vi "Construct.vi"(8 "error in (no error)":errorcluster, 9 "Ordered deps":refnum<class "ProjectItem.lvclass">[](array[class]), 10 "Application in":refnum<vi>, 11 "BuildManager in":refnum<class "BuildManager.lvclass">) -> (0 "error out":errorcluster, 3 "BuildManager out":refnum<class "BuildManager.lvclass">)   [LabVIEW 2020, in "SolutionBuilder.lvlib" / "BuildManager.lvclass"]
uses:
  BuildManager.lvclass
  ProjectItem/ProjectItem.lvclass
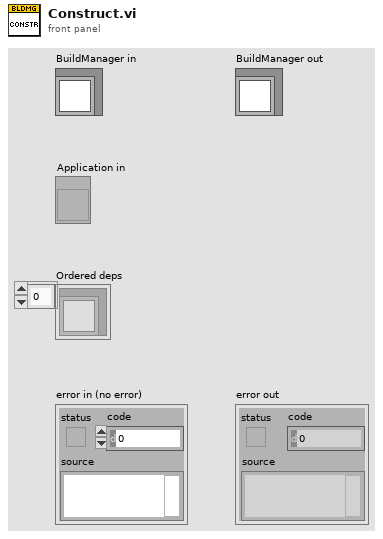
[diagram p1: front panel]
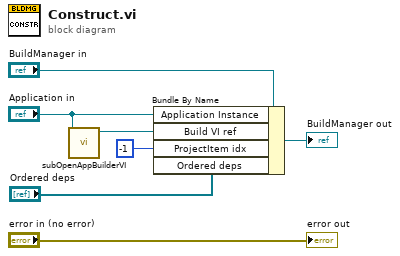
[diagram p0: block diagram]
diagram:
  n1 = call "subOpenAppBuilderVI.vi"("Application in"="Application in") -> ("VI ref"=w5:refnum<vi>)  [unwired: 10 in]
  n2 = Bundle By Name(cluster="BuildManager in", "Application Instance"="Application in", "Build VI ref"=w5, "ProjectItem idx"=-1, "Ordered deps"="Ordered deps") -> (→"BuildManager out":refnum<class "BuildManager.lvclass">)
  "error out" <- "error in (no error)"
